vi "Z Go.vi"(8 "error in (no error)":errorcluster, 9 "Speed":dbl format="%#_13g", 10 "Position":dbl format="%#_13g", 11 "Gantry In":refnum<k24>) -> (0 "error out":errorcluster, 3 "Gantry Out":refnum<k24>)   [LabVIEW 2020, in "A3200.lvclass"]
uses:
  A3200.lvclass
  C:/Program Files (x86)/Aerotech/A3200/LabVIEW/2010/Bin/Aerotech.A3200.dll
  Program Files (x86)/Aerotech/A3200/LabVIEW/2010/Bin/Aerotech.A3200.dll
  Drivers/Aerotech A3200/Aerotech VIs.lvlib
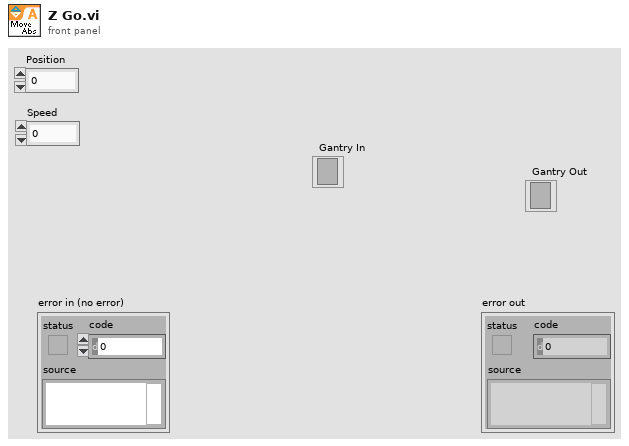
[diagram p1: front panel]
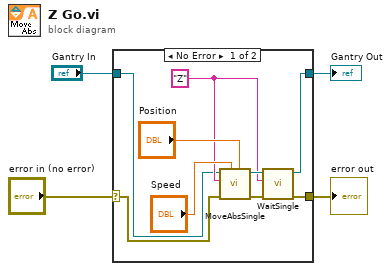
[diagram p0: block diagram]
diagram:
  n1 = case shown="No Error" "error in (no error)" {
    selector: "error in (no error)" -> [w8 w15]
    tunnel: [w6 w15] -> w3
    tunnel: "Gantry In" -> [w9 w14]
    tunnel: [w5 w14] -> w1
    frame No Error {
      w10 = "Z"
      n2 = call "MoveAbsSingle.vi"("position"="Position", "speed"="Speed", "error in (no error)"=w8, "axis name"=w10, "controller in"=w9) -> ("error out"=w7:errorcluster, "controller out"=w13:refnum<k24>)  [unwired: 5 in]
      n3 = call "WaitSingle.vi"("error in (no error)"=w7, "axis name"=w10, "controller in"=w13) -> ("error out"=w6:errorcluster, "controller out"=w5:refnum<k24>)  [unwired: 6 in, 1 out]
    }
    frame Error {
    }
  }
  "error out" <- w3
  "Gantry Out" <- w1
